vi "GetRTPCFlowsPressures.vi"(0 "Indices":i32[](array[numeric])) -> (1 "Flows":dbl[](array[numeric]), 2 "Pressures":dbl[](array[numeric]))   [LabVIEW 2011]
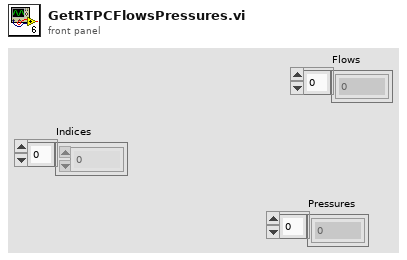
[diagram p1: front panel]
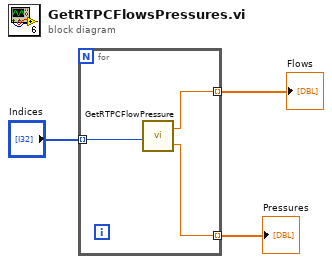
[diagram p0: block diagram]
diagram:
  n1 = for {
    tunnel: "Indices" -> [w6] mode=indexing
    tunnel: [w5] -> w2 mode=indexing
    tunnel: [w4] -> w1 mode=indexing
    n2 = call "GetRTPCFlowPressure.vi"("RTPC ID Number"=w6) -> ("Flow"=w5:dbl, "Pressure"=w4:dbl)
  }
  "Flows" <- w2
  "Pressures" <- w1
